vi "Sensor Data (Single Reading).vi"(8 "error in (no error)":errorcluster, 9 "Data Source (0:Kelvin)":u16(ring) items=["Kelvin", "Celsius", "Sensor Units"], 10 "Input (0:A)":u16(ring) items=["A", "B"], 11 "VISA resource name":refnum<visa-resource-name>) -> (0 "error out":errorcluster, 2 "Sensor Data":dbl format="%.4f", 3 "VISA resource name out":refnum<visa-resource-name>)   [LabVIEW 2012, in "Lake Shore 335.lvlib"]
doc: "Reads and returns a single sensor reading from the instrument."
uses:
  <instrlib>/lake shore 335/Temperature control panel Folder/C/Program Files/National Instruments/LabVIEW 2013/instr.lib/lake shore 335/Lake Shore 335.lvlib
  Instance           1 36Saved   Sensor Data (Single Reading) .vi
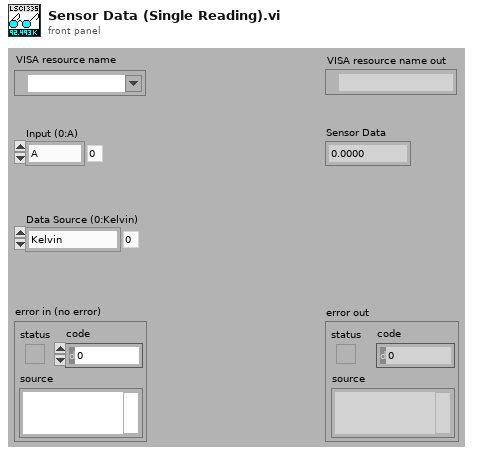
[diagram p1: front panel]
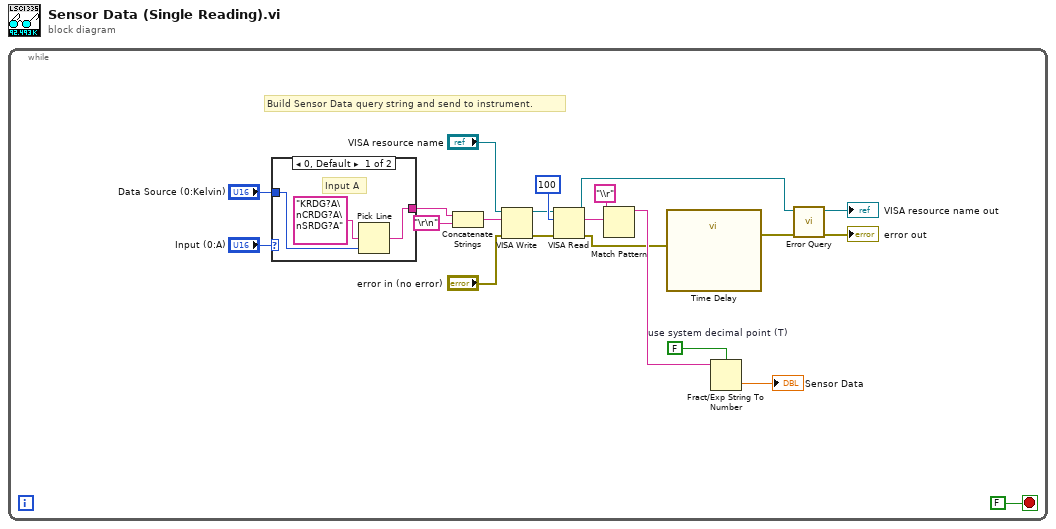
[diagram p0: block diagram]
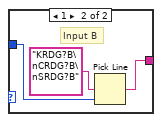
[diagram p2: hidden frame]
diagram:
  n1 = while {
    stop <- FALSE stop-if-true
    w11 = FALSE  # use system decimal point (T)
    # "Build Sensor Data query string and send to instrument."
    n2 = case shown="0, Default" "Input (0:A)" {
      tunnel: "Data Source (0:Kelvin)" -> [w23 w25]
      tunnel: [w22 w26] -> w2
      frame 0, Default {
        # "Input A"
        n3 = Pick Line(multi-line string="KRDG?A\nCRDG?A\nSRDG?A", line index=w23) -> (output string=w22:string)  [unwired: 1 in]
      }
      frame 1 {
        # "Input B"
        n4 = Pick Line(multi-line string="KRDG?B\nCRDG?B\nSRDG?B", line index=w25) -> (output string=w26:string)  [unwired: 1 in]
      }
    }
    n5 = Concatenate Strings(w2, "\r\n") -> (w3:string)
    n6 = VISA Write(VISA resource name="VISA resource name", write buffer=w3, error in (no error)="error in (no error)") -> (VISA resource name out=w13:refnum<visa-resource-name>, error out=w12:errorcluster)  [unwired: 1 out]
    n7 = VISA Read(VISA resource name=w13, byte count=100, error in (no error)=w12) -> (VISA resource name out=w17:refnum<visa-resource-name>, read buffer=w15:string, error out=w6:errorcluster)  [unwired: 1 out]
    n8 = Match Pattern(string=w15, regular expression="\\r") -> (before substring=w9:string)  [unwired: 1 in, 3 out]
    n9 = call "Time Delay"("error in (no error)"=w6) -> ("error out"=w7:errorcluster)  [unwired: 10 in]
    n10 = Fract/Exp String To Number(use system decimal point (T)=w11, string=w9) -> (number=→"Sensor Data":dbl)  [unwired: 2 in, 1 out]
    n11 = call <instrlib>:"Error Query.vi"("error in (no error)"=w7, "VISA resource name"=w17) -> ("error out"=→"error out":errorcluster, "VISA resource name out"=→"VISA resource name out":refnum<visa-resource-name>)  [unwired: 7 in, 1 out]
  }
